vi "run_plot_graph.vi"(0 "xValues":i32, 1 "yValues":i32, 2 "File Path":path, 3 "xName":string, 4 "yName":string) -> ()   [LabVIEW 2019]
uses:
  <vilib>/Analysis/Matrix/Numeric/Conversions/Array To Matrix - RA2.vi
  <vilib>/Analysis/Matrix/Numeric/Conversions/Matrix To Array - RM.vi
  <vilib>/Analysis/Matrix/NI_Matrix.lvlib
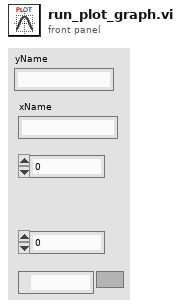
[diagram p1: front panel]
types:
  T1 = typedef "NI_Matrix.lvlib/RealMatrix.ctl" = dbl[][]
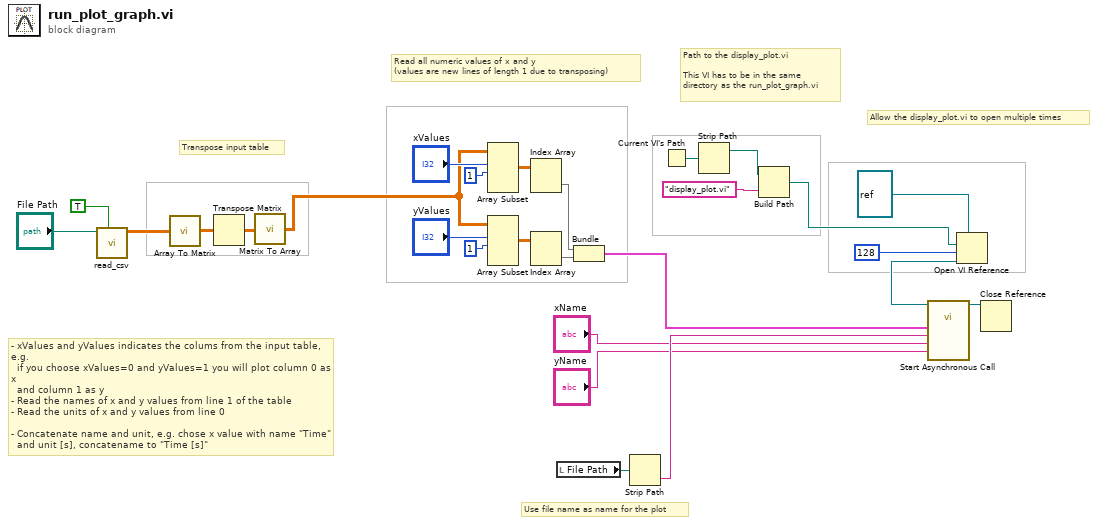
[diagram p0: block diagram]
diagram:
  # "Path to the display_plot.vi\n\nThis VI has to be in the same \ndirectory as the run_plot_graph.vi"
  # "Allow the display_plot.vi to open multiple times"
  # "Use file name as name for the plot"
  # "Read all numeric values of x and y\n(values are new lines of length 1 due to transposing)"
  # "Transpose input table"
  # "- xValues and yValues indicates the colums from the input table, e.g.\n  if you choose xValues=0 and yValues=1 you will plot column 0 as x \n  and column 1 as y\n- Read the names of x and y values from line 1 of the table\n- Read the units of x and y values from line 0\n\n- Concatenate name and unit, e.g. chose x value with name \"Time\"\n  and unit [s], concatename to \"Time [s]\""
  n1 = call "read_csv.vi"("Read"=TRUE, "Read File:"="File Path") -> ("File Data"=w12:T1)  [unwired: 7 in, 2 out]
  n2 = call-poly <vilib>:"Array To Matrix.vi"("Real 2D Array"=w12) -> ("Real Matrix"=w21:T1)
  n3 = Transpose Matrix(1:w21) -> (0:w22:T1)
  n4 = call-poly <vilib>:"Matrix To Array.vi"("Real Matrix"=w22) -> ("Real 2D Array"=w18:dbl[][])
  n5 = Array Subset(array=w18, index (row)="xValues", length (row)=1 ("length")) -> (w17:dbl[][])  [unwired: 2 in]
  n6 = Array Subset(array=w18, index (row)="yValues", length (row)=1 ("length")) -> (w15:dbl[][])  [unwired: 2 in]
  n7 = Index Array(array=w17) -> (element=w16:dbl[])  [unwired: 2 in]
  n8 = Index Array(array=w15) -> (element=w14:dbl[])  [unwired: 2 in]
  n9 = local read "File Path"() -> (w8:path)
  n10 = Bundle(w16, w14) -> (w26:cluster{dbl[], dbl[]})  [unwired: 1 in]
  n11 = Strip Path(path=w8) -> (name=w7:string)  [unwired: 1 out]
  n12 = Current VI's Path() -> (path=w4:path)
  n13 = Strip Path(path=w4) -> (stripped path=w3:path)  [unwired: 1 out]
  n14 = Build Path(base path=w3, name or relative path="display_plot.vi" ("string")) -> (appended path=w5:path)
  n15 = Open VI Reference(type specifier VI Refnum (for type only)=refnum<vi> refnum, vi path=w5, options=128) -> (vi reference=w27:refnum<vi>)  [unwired: 3 in, 1 out]
  n16 = call-by-ref "Start Asynchronous Call"(reference=w27, "Y Scale.Name Label.Text"="yName", "X Scale.Name Label.Text"="xName", "FileName"=w7, "Input Data"=w26) -> (reference out=w25:refnum<vi>)  [unwired: 9 in, 1 out]
  n17 = Close Reference(reference=w25) -> ()  [unwired: 1 in, 1 out]
